vi "Constants.vi"() -> ()   [LabVIEW 2017]
panel:
  in  "CenterRotOffset":dbl=10.25
  in  "Height":dbl=29.0
  in  "Width":dbl=32.0
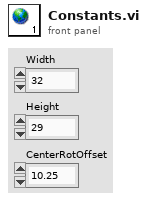
[diagram p1: front panel]
diagram:
